vi "GetMac.vi"(8 "error in (no error)":errorcluster caption="错误输入（无错误）", 9 "Password":string caption="密码", 10 "User Name":string caption="用户名", 11 "Target":refnum<k21>="localhost" caption="终端") -> (0 "error out":errorcluster caption="错误输出", 1 "网络适配器:MAC地址":string)   [LabVIEW 2018]
uses:
  <vilib>/nisyscfg/Close (Filter).vi
  <vilib>/nisyscfg/Close (System).vi
  <vilib>/nisyscfg/nisyscfg.lvlib
  <resource>/objmgr/nisysapi.rc
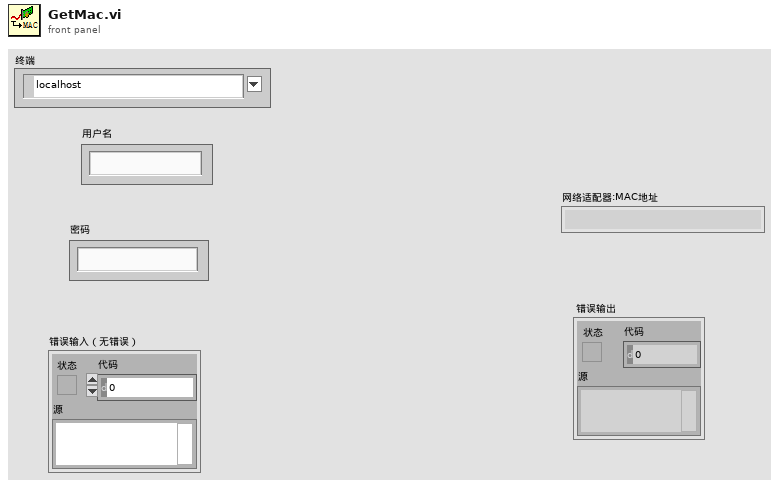
[diagram p1: front panel]
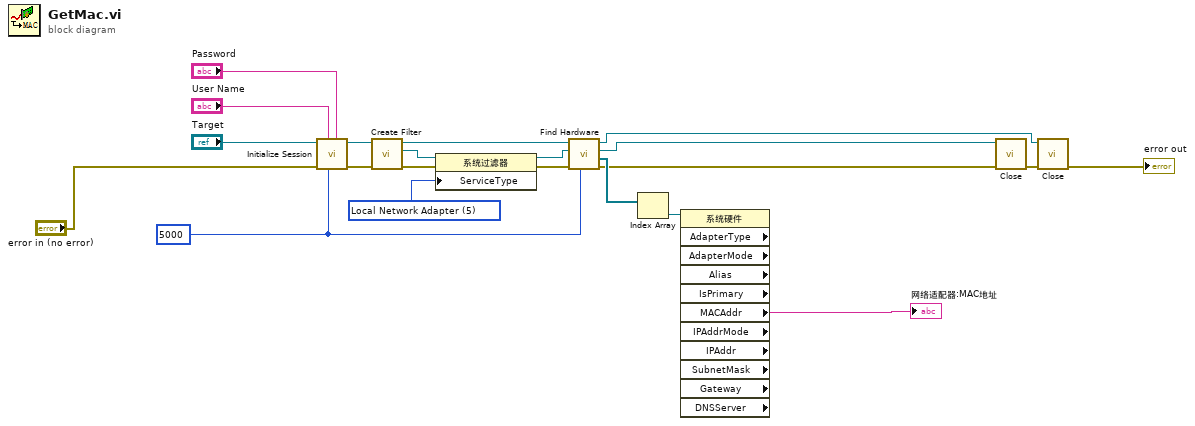
[diagram p0: block diagram]
diagram:
  w11 = u32 5000 ("Timeout (milliseconds)")
  w10 = u32 5 items=["NI Network Resource", "NI Real-Time", "NI System Configuration", "NI Web Interface", "Local System", "Local Network Adapter", "Local Time Keeper", "Local Time Reference", "LXI Instrument"] ("Service Type")
  n1 = call <vilib>:"Initialize Session.vi"("Password"="Password", "Connect Timeout (4000 ms)"=w11, "User Name"="User Name", "error in (no error)"="error in (no error)", "Target (localhost)"="Target") -> ("error out"=w20:errorcluster, "Session out"=w21:refnum<k21>)  [unwired: 5 in]
  n2 = call <vilib>:"Create Filter.vi"("error in (no error)"=w20, "Session in"=w21) -> ("error out"=w18:errorcluster, "Filter out"=w19:refnum<k20>, "Session out"=w16:refnum<k21>)  [unwired: 7 in]
  n3 = property class="系统过滤器"(reference=w19, error in=w18, "ServiceType"=w10) -> (reference out=w15:refnum<k20>, error out=w17:errorcluster)
  n4 = call <vilib>:"Find Hardware.vi"("Remote Timeout (300,000 ms)"=w11, "error in (no error)"=w17, "Filter in"=w15, "Session in"=w16) -> ("error out"=w4:errorcluster, "Resources out"=w9:refnum<k20>[], "Filter out"=w6:refnum<k20>, "Session out"=w5:refnum<k21>)  [unwired: 4 in]
  n5 = Index Array(array=w9) -> (element=w8:refnum<k20>)  [unwired: 1 in]
  n6 = property class="系统硬件" props=["AdapterType", "AdapterMode", "Alias", "IsPrimary", "MACAddr", "IPAddrMode", "IPAddr", "SubnetMask", "Gateway", "DNSServer"](reference=w8) -> ("MACAddr"=→"网络适配器:MAC地址":string)  [unwired: 1 in, 11 out]
  n7 = call-poly <vilib>:"Close.vi"("error in (no error)"=w4, "Filter in"=w6) -> ("error out"=w7:errorcluster)  [unwired: 9 in]
  n8 = call-poly <vilib>:"Close.vi"("error in (no error)"=w7, "Session in"=w5) -> ("error out"=→"error out":errorcluster)  [unwired: 9 in]
